vi "TesterOption (SubVI).vi"(5 "On/Off 2":bool=TRUE, 6 "Tester Option 2":T1(ring), 7 "2 Options":bool, 8 "error in (no error)":errorcluster, 9 "On/Off":bool=TRUE, 10 "Tester Option":T1(ring), 11 "VISA Refnum in":refnum<visa-resource-name>) -> (0 "error out":errorcluster, 3 "VISA Refnum out":refnum<visa-resource-name>)   [LabVIEW 2017]
panel:
  out "x .or. y?":u8[](array[numeric])
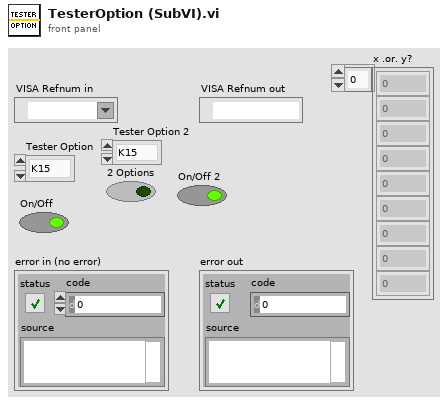
[diagram p1: front panel]
types:
  T1 = enum16{"K15", "K16", "K17", "Venable", "Firmeware", "Fan", "Power", "120C", "110C", "100C", "90C", "80C", "70C", "60C", "50C", "40C", "30C", "25C", "20C", "10C", "0C"}
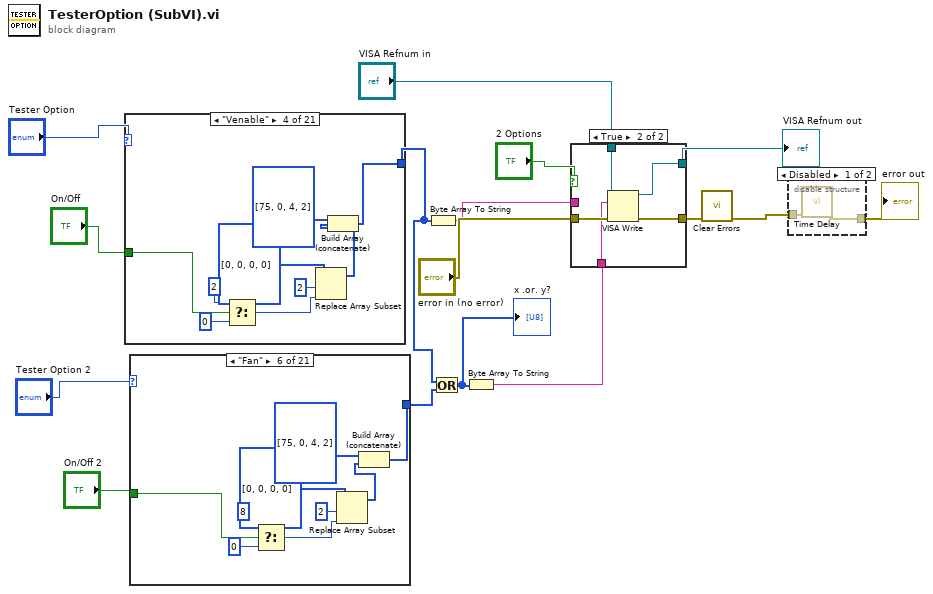
[diagram p0: block diagram]
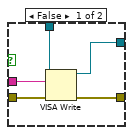
[diagram p3: hidden frame]
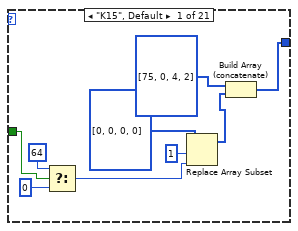
[diagram p4: hidden frame]
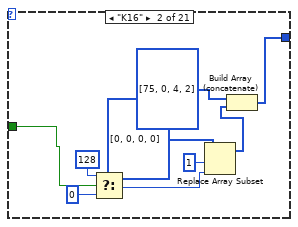
[diagram p5: hidden frame]
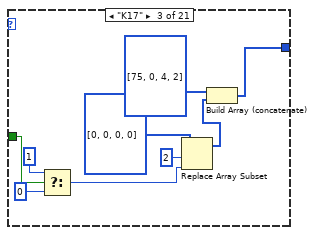
[diagram p6: hidden frame]
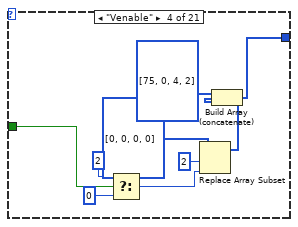
[diagram p7: hidden frame]
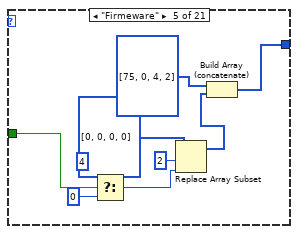
[diagram p8: hidden frame]
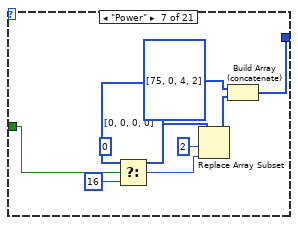
[diagram p9: hidden frame]
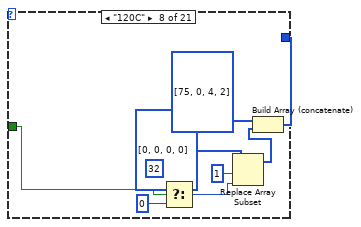
[diagram p10: hidden frame]
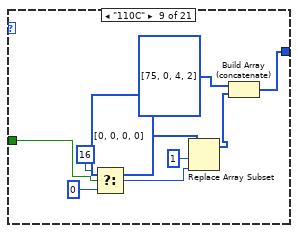
[diagram p11: hidden frame]
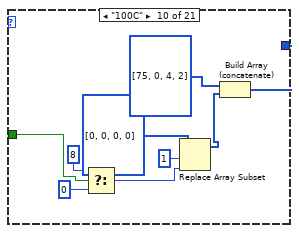
[diagram p12: hidden frame]
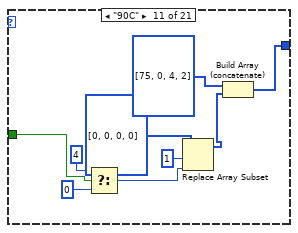
[diagram p13: hidden frame]
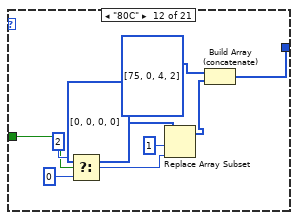
[diagram p14: hidden frame]
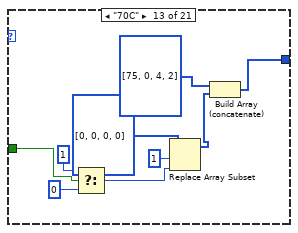
[diagram p15: hidden frame]
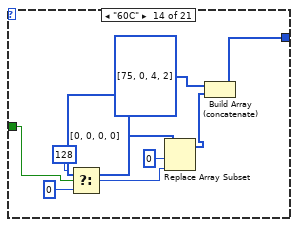
[diagram p16: hidden frame]
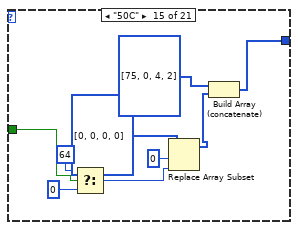
[diagram p17: hidden frame]
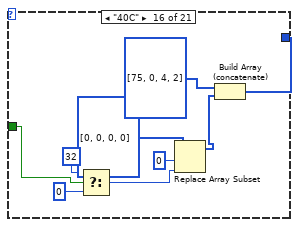
[diagram p18: hidden frame]
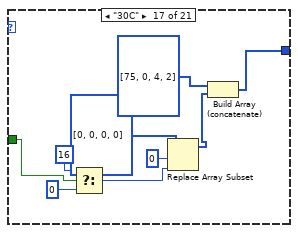
[diagram p19: hidden frame]
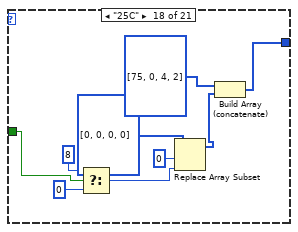
[diagram p20: hidden frame]
diagram:
  n1 = case shown="\"Venable\"" "Tester Option" {
    tunnel: [w24 w33 w35 w51 w60 w69 w77 w81 w89 w99 w108 w117 w125 w135 w144 w153 w162 w171 w180 w189 w198] -> w4
    tunnel: "On/Off" -> [w18 w27 w36 w45 w54 w63 w73 w80 w90 w98 w107 w116 w126 w134 w143 w152 w161 w170 w179 w188 w197]
    frame "K15", Default {
      n2 = Select(t=u8 64, s=w18, f=u8 0) -> (s? t:f=w19:u8)
      n3 = Replace Array Subset(array=u8[] [0, 0, 0, 0], new element=w19, index=1) -> (w17:u8[])
      n4 = Build Array (concatenate)(u8[] [75, 0, 4, 2], w17) -> (w24:u8[])
    }
    frame "K16" {
      n5 = Select(t=u8 128, s=w27, f=u8 0) -> (s? t:f=w28:u8)
      n6 = Replace Array Subset(array=u8[] [0, 0, 0, 0], new element=w28, index=1) -> (w26:u8[])
      n7 = Build Array (concatenate)(u8[] [75, 0, 4, 2], w26) -> (w33:u8[])
    }
    frame "K17" {
      n8 = Select(t=u8 1, s=w36, f=u8 0) -> (s? t:f=w38:u8)
      n9 = Replace Array Subset(array=u8[] [0, 0, 0, 0], new element=w38, index=2) -> (w37:u8[])
      n10 = Build Array (concatenate)(u8[] [75, 0, 4, 2], w37) -> (w35:u8[])
    }
    frame "Venable" {
      n11 = Select(t=u8 2, s=w45, f=u8 0) -> (s? t:f=w46:u8)
      n12 = Replace Array Subset(array=u8[] [0, 0, 0, 0], new element=w46, index=2) -> (w44:u8[])
      n13 = Build Array (concatenate)(u8[] [75, 0, 4, 2], w44) -> (w51:u8[])
    }
    frame "Firmeware" {
      n14 = Select(t=u8 4, s=w54, f=u8 0) -> (s? t:f=w55:u8)
      n15 = Replace Array Subset(array=u8[] [0, 0, 0, 0], new element=w55, index=2) -> (w53:u8[])
      n16 = Build Array (concatenate)(u8[] [75, 0, 4, 2], w53) -> (w60:u8[])
    }
    frame "Fan" {
      n17 = Select(t=u8 8, s=w63, f=u8 0) -> (s? t:f=w64:u8)
      n18 = Replace Array Subset(array=u8[] [0, 0, 0, 0], new element=w64, index=2) -> (w62:u8[])
      n19 = Build Array (concatenate)(u8[] [75, 0, 4, 2], w62) -> (w69:u8[])
    }
    frame "Power" {
      n20 = Select(t=u8 0, s=w73, f=u8 16) -> (s? t:f=w71:u8)
      n21 = Replace Array Subset(array=u8[] [0, 0, 0, 0], new element=w71, index=2) -> (w76:u8[])
      n22 = Build Array (concatenate)(u8[] [75, 0, 4, 2], w76) -> (w77:u8[])
    }
    frame "120C" {
      n23 = Select(t=u8 32, s=w80, f=u8 0) -> (s? t:f=w83:u8)
      n24 = Replace Array Subset(array=u8[] [0, 0, 0, 0], new element=w83, index=1) -> (w82:u8[])
      n25 = Build Array (concatenate)(u8[] [75, 0, 4, 2], w82) -> (w81:u8[])
    }
    frame "110C" {
      n26 = Select(t=u8 16, s=w90, f=u8 0) -> (s? t:f=w92:u8)
      n27 = Replace Array Subset(array=u8[] [0, 0, 0, 0], new element=w92, index=1) -> (w91:u8[])
      n28 = Build Array (concatenate)(u8[] [75, 0, 4, 2], w91) -> (w89:u8[])
    }
    frame "100C" {
      n29 = Select(t=u8 8, s=w98, f=u8 0) -> (s? t:f=w101:u8)
      n30 = Replace Array Subset(array=u8[] [0, 0, 0, 0], new element=w101, index=1) -> (w100:u8[])
      n31 = Build Array (concatenate)(u8[] [75, 0, 4, 2], w100) -> (w99:u8[])
    }
    frame "90C" {
      n32 = Select(t=u8 4, s=w107, f=u8 0) -> (s? t:f=w110:u8)
      n33 = Replace Array Subset(array=u8[] [0, 0, 0, 0], new element=w110, index=1) -> (w109:u8[])
      n34 = Build Array (concatenate)(u8[] [75, 0, 4, 2], w109) -> (w108:u8[])
    }
    frame "80C" {
      n35 = Select(t=u8 2, s=w116, f=u8 0) -> (s? t:f=w119:u8)
      n36 = Replace Array Subset(array=u8[] [0, 0, 0, 0], new element=w119, index=1) -> (w118:u8[])
      n37 = Build Array (concatenate)(u8[] [75, 0, 4, 2], w118) -> (w117:u8[])
    }
    frame "70C" {
      n38 = Select(t=u8 1, s=w126, f=u8 0) -> (s? t:f=w128:u8)
      n39 = Replace Array Subset(array=u8[] [0, 0, 0, 0], new element=w128, index=1) -> (w127:u8[])
      n40 = Build Array (concatenate)(u8[] [75, 0, 4, 2], w127) -> (w125:u8[])
    }
    frame "60C" {
      n41 = Select(t=u8 128, s=w134, f=u8 0) -> (s? t:f=w137:u8)
      n42 = Replace Array Subset(array=u8[] [0, 0, 0, 0], new element=w137, index=0) -> (w136:u8[])
      n43 = Build Array (concatenate)(u8[] [75, 0, 4, 2], w136) -> (w135:u8[])
    }
    frame "50C" {
      n44 = Select(t=u8 64, s=w143, f=u8 0) -> (s? t:f=w146:u8)
      n45 = Replace Array Subset(array=u8[] [0, 0, 0, 0], new element=w146, index=0) -> (w145:u8[])
      n46 = Build Array (concatenate)(u8[] [75, 0, 4, 2], w145) -> (w144:u8[])
    }
    frame "40C" {
      n47 = Select(t=u8 32, s=w152, f=u8 0) -> (s? t:f=w155:u8)
      n48 = Replace Array Subset(array=u8[] [0, 0, 0, 0], new element=w155, index=0) -> (w154:u8[])
      n49 = Build Array (concatenate)(u8[] [75, 0, 4, 2], w154) -> (w153:u8[])
    }
    frame "30C" {
      n50 = Select(t=u8 16, s=w161, f=u8 0) -> (s? t:f=w164:u8)
      n51 = Replace Array Subset(array=u8[] [0, 0, 0, 0], new element=w164, index=0) -> (w163:u8[])
      n52 = Build Array (concatenate)(u8[] [75, 0, 4, 2], w163) -> (w162:u8[])
    }
    frame "25C" {
      n53 = Select(t=u8 8, s=w170, f=u8 0) -> (s? t:f=w173:u8)
      n54 = Replace Array Subset(array=u8[] [0, 0, 0, 0], new element=w173, index=0) -> (w172:u8[])
      n55 = Build Array (concatenate)(u8[] [75, 0, 4, 2], w172) -> (w171:u8[])
    }
    frame "20C" {
      n56 = Select(t=u8 4, s=w179, f=u8 0) -> (s? t:f=w182:u8)
      n57 = Replace Array Subset(array=u8[] [0, 0, 0, 0], new element=w182, index=0) -> (w181:u8[])
      n58 = Build Array (concatenate)(u8[] [75, 0, 4, 2], w181) -> (w180:u8[])
    }
    frame "10C" {
      n59 = Select(t=u8 2, s=w188, f=u8 0) -> (s? t:f=w191:u8)
      n60 = Replace Array Subset(array=u8[] [0, 0, 0, 0], new element=w191, index=0) -> (w190:u8[])
      n61 = Build Array (concatenate)(u8[] [75, 0, 4, 2], w190) -> (w189:u8[])
    }
    frame "0C" {
      n62 = Select(t=u8 1, s=w197, f=u8 0) -> (s? t:f=w200:u8)
      n63 = Replace Array Subset(array=u8[] [0, 0, 0, 0], new element=w200, index=0) -> (w199:u8[])
      n64 = Build Array (concatenate)(u8[] [75, 0, 4, 2], w199) -> (w198:u8[])
    }
  }
  n65 = case shown="\"Fan\"" "Tester Option 2" {
    tunnel: [w213 w222 w224 w240 w249 w258 w266 w269 w279 w288 w297 w306 w314 w324 w333 w342 w351 w360 w369 w378 w387] -> w7
    tunnel: "On/Off 2" -> [w207 w216 w225 w234 w243 w252 w262 w270 w278 w287 w296 w305 w315 w323 w332 w341 w350 w359 w368 w377 w386]
    frame "K15", Default {
      n66 = Select(t=u8 64, s=w207, f=u8 0) -> (s? t:f=w208:u8)
      n67 = Replace Array Subset(array=u8[] [0, 0, 0, 0], new element=w208, index=1) -> (w206:u8[])
      n68 = Build Array (concatenate)(u8[] [75, 0, 4, 2], w206) -> (w213:u8[])
    }
    frame "K16" {
      n69 = Select(t=u8 128, s=w216, f=u8 0) -> (s? t:f=w217:u8)
      n70 = Replace Array Subset(array=u8[] [0, 0, 0, 0], new element=w217, index=1) -> (w215:u8[])
      n71 = Build Array (concatenate)(u8[] [75, 0, 4, 2], w215) -> (w222:u8[])
    }
    frame "K17" {
      n72 = Select(t=u8 1, s=w225, f=u8 0) -> (s? t:f=w227:u8)
      n73 = Replace Array Subset(array=u8[] [0, 0, 0, 0], new element=w227, index=2) -> (w226:u8[])
      n74 = Build Array (concatenate)(u8[] [75, 0, 4, 2], w226) -> (w224:u8[])
    }
    frame "Venable" {
      n75 = Select(t=u8 2, s=w234, f=u8 0) -> (s? t:f=w235:u8)
      n76 = Replace Array Subset(array=u8[] [0, 0, 0, 0], new element=w235, index=2) -> (w233:u8[])
      n77 = Build Array (concatenate)(u8[] [75, 0, 4, 2], w233) -> (w240:u8[])
    }
    frame "Firmeware" {
      n78 = Select(t=u8 4, s=w243, f=u8 0) -> (s? t:f=w244:u8)
      n79 = Replace Array Subset(array=u8[] [0, 0, 0, 0], new element=w244, index=2) -> (w242:u8[])
      n80 = Build Array (concatenate)(u8[] [75, 0, 4, 2], w242) -> (w249:u8[])
    }
    frame "Fan" {
      n81 = Select(t=u8 8, s=w252, f=u8 0) -> (s? t:f=w253:u8)
      n82 = Replace Array Subset(array=u8[] [0, 0, 0, 0], new element=w253, index=2) -> (w251:u8[])
      n83 = Build Array (concatenate)(u8[] [75, 0, 4, 2], w251) -> (w258:u8[])
    }
    frame "Power" {
      n84 = Select(t=u8 0, s=w262, f=u8 16) -> (s? t:f=w260:u8)
      n85 = Replace Array Subset(array=u8[] [0, 0, 0, 0], new element=w260, index=2) -> (w265:u8[])
      n86 = Build Array (concatenate)(u8[] [75, 0, 4, 2], w265) -> (w266:u8[])
    }
    frame "120C" {
      n87 = Select(t=u8 32, s=w270, f=u8 0) -> (s? t:f=w272:u8)
      n88 = Replace Array Subset(array=u8[] [0, 0, 0, 0], new element=w272, index=1) -> (w271:u8[])
      n89 = Build Array (concatenate)(u8[] [75, 0, 4, 2], w271) -> (w269:u8[])
    }
    frame "110C" {
      n90 = Select(t=u8 16, s=w278, f=u8 0) -> (s? t:f=w281:u8)
      n91 = Replace Array Subset(array=u8[] [0, 0, 0, 0], new element=w281, index=1) -> (w280:u8[])
      n92 = Build Array (concatenate)(u8[] [75, 0, 4, 2], w280) -> (w279:u8[])
    }
    frame "100C" {
      n93 = Select(t=u8 8, s=w287, f=u8 0) -> (s? t:f=w290:u8)
      n94 = Replace Array Subset(array=u8[] [0, 0, 0, 0], new element=w290, index=1) -> (w289:u8[])
      n95 = Build Array (concatenate)(u8[] [75, 0, 4, 2], w289) -> (w288:u8[])
    }
    frame "90C" {
      n96 = Select(t=u8 4, s=w296, f=u8 0) -> (s? t:f=w299:u8)
      n97 = Replace Array Subset(array=u8[] [0, 0, 0, 0], new element=w299, index=1) -> (w298:u8[])
      n98 = Build Array (concatenate)(u8[] [75, 0, 4, 2], w298) -> (w297:u8[])
    }
    frame "80C" {
      n99 = Select(t=u8 2, s=w305, f=u8 0) -> (s? t:f=w308:u8)
      n100 = Replace Array Subset(array=u8[] [0, 0, 0, 0], new element=w308, index=1) -> (w307:u8[])
      n101 = Build Array (concatenate)(u8[] [75, 0, 4, 2], w307) -> (w306:u8[])
    }
    frame "70C" {
      n102 = Select(t=u8 1, s=w315, f=u8 0) -> (s? t:f=w317:u8)
      n103 = Replace Array Subset(array=u8[] [0, 0, 0, 0], new element=w317, index=1) -> (w316:u8[])
      n104 = Build Array (concatenate)(u8[] [75, 0, 4, 2], w316) -> (w314:u8[])
    }
    frame "60C" {
      n105 = Select(t=u8 128, s=w323, f=u8 0) -> (s? t:f=w326:u8)
      n106 = Replace Array Subset(array=u8[] [0, 0, 0, 0], new element=w326, index=0) -> (w325:u8[])
      n107 = Build Array (concatenate)(u8[] [75, 0, 4, 2], w325) -> (w324:u8[])
    }
    frame "50C" {
      n108 = Select(t=u8 64, s=w332, f=u8 0) -> (s? t:f=w335:u8)
      n109 = Replace Array Subset(array=u8[] [0, 0, 0, 0], new element=w335, index=0) -> (w334:u8[])
      n110 = Build Array (concatenate)(u8[] [75, 0, 4, 2], w334) -> (w333:u8[])
    }
    frame "40C" {
      n111 = Select(t=u8 32, s=w341, f=u8 0) -> (s? t:f=w344:u8)
      n112 = Replace Array Subset(array=u8[] [0, 0, 0, 0], new element=w344, index=0) -> (w343:u8[])
      n113 = Build Array (concatenate)(u8[] [75, 0, 4, 2], w343) -> (w342:u8[])
    }
    frame "30C" {
      n114 = Select(t=u8 16, s=w350, f=u8 0) -> (s? t:f=w353:u8)
      n115 = Replace Array Subset(array=u8[] [0, 0, 0, 0], new element=w353, index=0) -> (w352:u8[])
      n116 = Build Array (concatenate)(u8[] [75, 0, 4, 2], w352) -> (w351:u8[])
    }
    frame "25C" {
      n117 = Select(t=u8 8, s=w359, f=u8 0) -> (s? t:f=w362:u8)
      n118 = Replace Array Subset(array=u8[] [0, 0, 0, 0], new element=w362, index=0) -> (w361:u8[])
      n119 = Build Array (concatenate)(u8[] [75, 0, 4, 2], w361) -> (w360:u8[])
    }
    frame "20C" {
      n120 = Select(t=u8 4, s=w368, f=u8 0) -> (s? t:f=w371:u8)
      n121 = Replace Array Subset(array=u8[] [0, 0, 0, 0], new element=w371, index=0) -> (w370:u8[])
      n122 = Build Array (concatenate)(u8[] [75, 0, 4, 2], w370) -> (w369:u8[])
    }
    frame "10C" {
      n123 = Select(t=u8 2, s=w377, f=u8 0) -> (s? t:f=w380:u8)
      n124 = Replace Array Subset(array=u8[] [0, 0, 0, 0], new element=w380, index=0) -> (w379:u8[])
      n125 = Build Array (concatenate)(u8[] [75, 0, 4, 2], w379) -> (w378:u8[])
    }
    frame "0C" {
      n126 = Select(t=u8 1, s=w386, f=u8 0) -> (s? t:f=w389:u8)
      n127 = Replace Array Subset(array=u8[] [0, 0, 0, 0], new element=w389, index=0) -> (w388:u8[])
      n128 = Build Array (concatenate)(u8[] [75, 0, 4, 2], w388) -> (w387:u8[])
    }
  }
  n129 = Byte Array To String(unsigned byte array=w4) -> (string=w12:string)
  n130 = Or(x=w4, y=w7) -> (x .or. y?=w2:u8[])
  "x .or. y?" <- w2
  n131 = Byte Array To String(unsigned byte array=w2) -> (string=w5:string)
  n132 = case shown="True" "2 Options" {
    tunnel: [w399 w404] -> w16
    tunnel: "error in (no error)" -> [w398 w403]
    tunnel: [w397 w402] -> w14
    tunnel: "VISA Refnum in" -> [w396 w401]
    tunnel: w12 -> [w395 _]
    tunnel: w5 -> [_ w400]
    frame False {
      n133 = VISA Write(VISA resource name=w396, write buffer=w395, error in (no error)=w398) -> (VISA resource name out=w397:refnum<visa-resource-name>, error out=w399:errorcluster)  [unwired: 1 out]
    }
    frame True {
      n134 = VISA Write(VISA resource name=w401, write buffer=w400, error in (no error)=w403) -> (VISA resource name out=w402:refnum<visa-resource-name>, error out=w404:errorcluster)  [unwired: 1 out]
    }
  }
  "VISA Refnum out" <- w14
  n135 = call <vilib>:"Clear Errors.vi"("error in (no error)"=w16) -> ("error out"=w3:errorcluster)  [unwired: 5 in, 1 out]
  n136 = disable-structure shown="Disabled" {
    disable-tunnel: w3 -> [w406 w407]
    disable-tunnel: [w405 w407] -> w1
    frame Disabled {
      n137 = call "Time Delay"("error in (no error)"=w406) -> ("error out"=w405:errorcluster)  [unwired: 10 in]
    }
    frame Enabled {
    }
  }
  "error out" <- w1
